vi "Asylum_ShowVideo.vi"(8 "error in (no error)":errorcluster, 10 "Source":i32, 11 "Application":refnum<k7>) -> (0 "error out":errorcluster, 3 "Application":refnum<k7>)   [LabVIEW 2020]
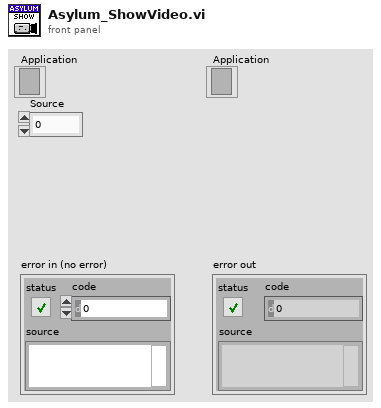
[diagram p1: front panel]
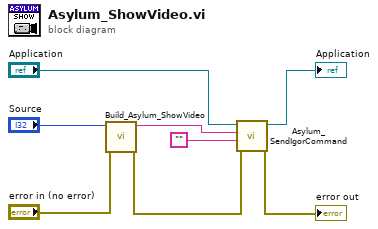
[diagram p0: block diagram]
diagram:
  n1 = call "Build_Asylum_ShowVideo.vi"("error in (no error)"="error in (no error)", "Source"="Source") -> ("error out"=w8:errorcluster, "Command"=w6:string)  [unwired: 8 in]
  n2 = call "Asylum_SendIgorCommand.vi"("error in (no error)"=w8, "Format"="", "command"=w6, "Application"="Application") -> ("error out"=→"error out":errorcluster, "Application"=→"Application":refnum<k7>)  [unwired: 4 in, 2 out]
